vi "XYQuickView.vi"(9 "listOfProfiles":path[](array[path])) -> ()   [LabVIEW 2014]
uses:
  <vilib>/Utility/file.llb/Read From Spreadsheet File (DBL).vi
panel:
  out "XY Graph":cluster{"Y":dbl[], "Y":dbl[]}[](graph)
  in  "fileDelimiter":u16(ring) items=["tab", "space", "comma"]
  in  "open files":bool
  in  "plotType":u16(ring) items=["symbols", "line", "line+symbols"]
  in  "stop":bool
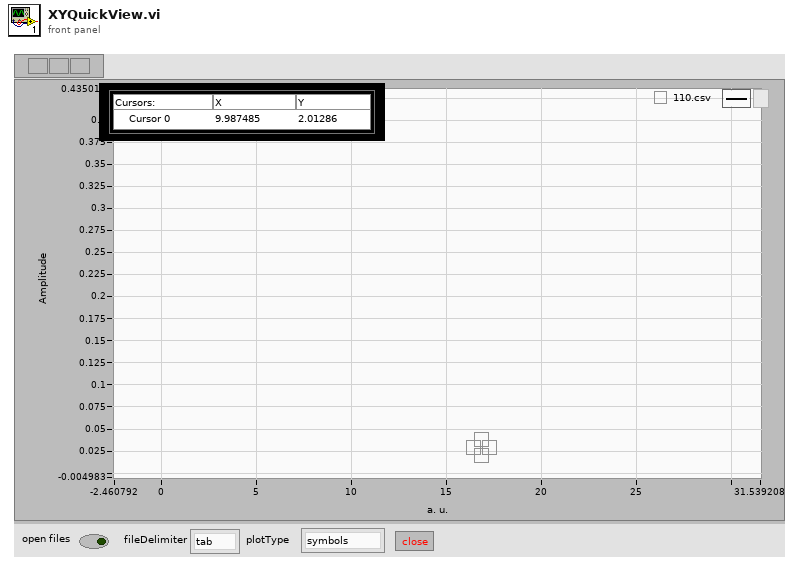
[diagram p1: front panel]
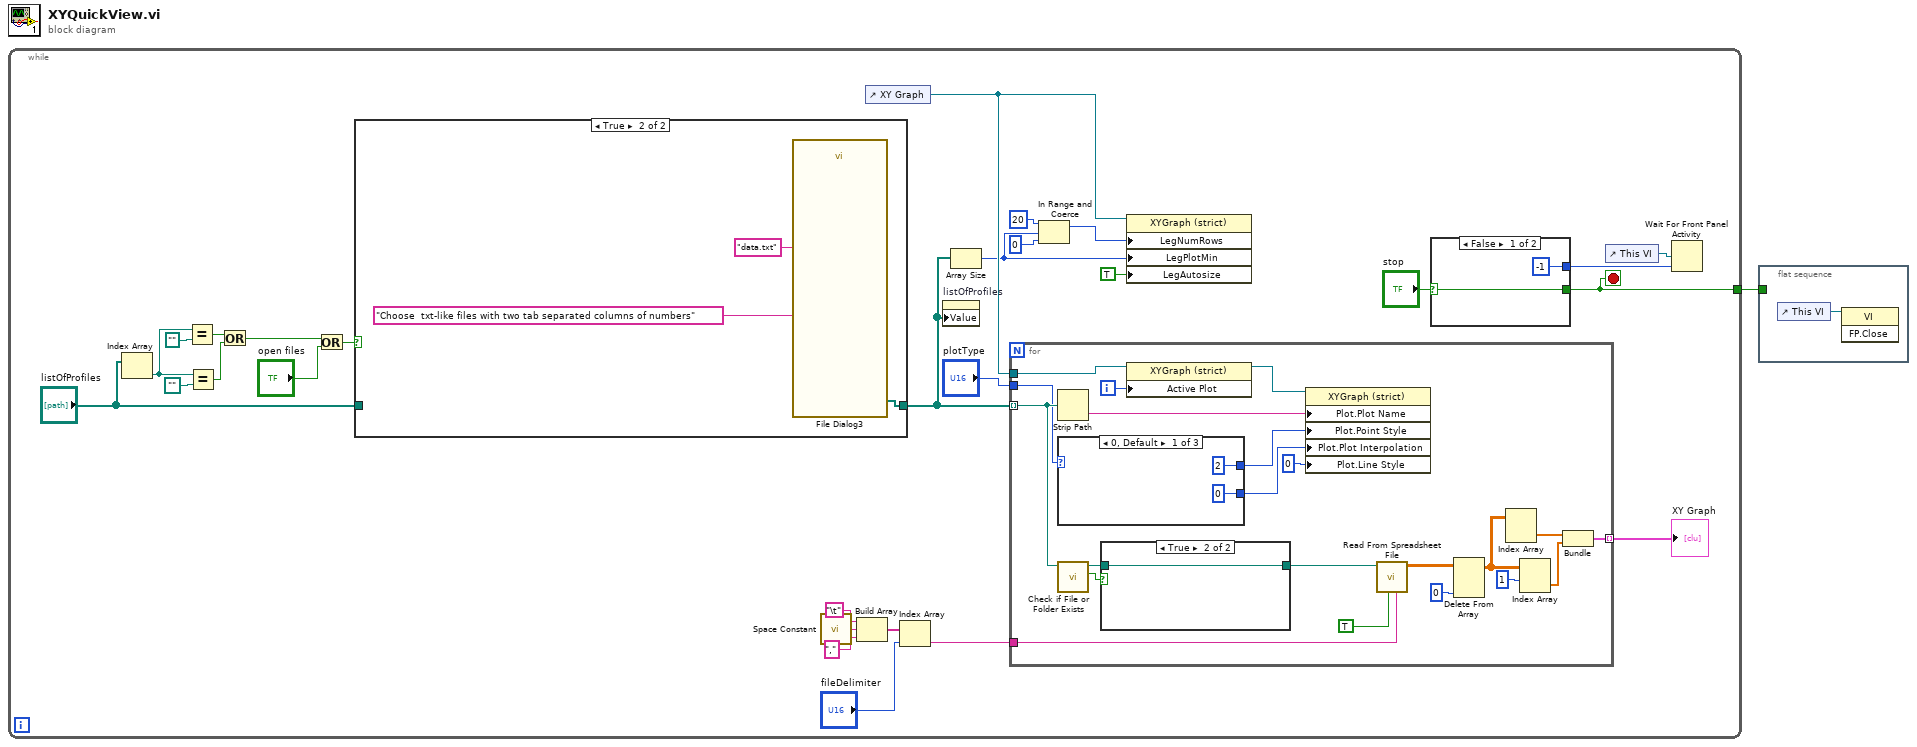
[diagram p0: block diagram]
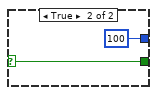
[diagram p3: hidden frame]
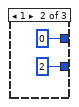
[diagram p4: hidden frame]
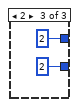
[diagram p5: hidden frame]
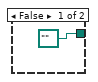
[diagram p6: hidden frame]
diagram:
  n1 = while {
    tunnel: [w17] -> w1
    stop <- w17 stop-if-true
    n2 = Index Array(array="listOfProfiles") -> (element=w20:path)  [unwired: 1 in]
    n3 = Equal?(x=w20, y=path "") -> (x = y?=w22:bool)
    n4 = Equal?(x=w20, y=path "") -> (x = y?=w21:bool)
    n5 = Or(x=w22, y=w21) -> (x .or. y?=w16:bool)
    n6 = Or(x=w16, y="open files") -> (x .or. y?=w14:bool)
    n7 = case shown="True" w14 {
      tunnel: [w30 w31] -> w18
      tunnel: "listOfProfiles" -> [w30 _]
      frame False {
      }
      frame True {
        n8 = call "File Dialog3"("prompt"="Choose  txt-like files with two tab separated columns of numbers" ("Prompt"), "default name"="data.txt") -> ("selected paths"=w31:path[])  [unwired: 10 in, 3 out]
      }
    }
    n9 = call <vilib>:"Space Constant.vi"() -> ("String"=w7:string)
    n10 = Build Array("\t", w7, ",") -> (w11:string[])
    n11 = control-ref of="XY Graph"() -> (w29:refnum<vi>)
    n12 = Index Array(array=w11, index="fileDelimiter") -> (element=w9:string)
    n13 = property on="listOfProfiles" class="Arr (strict)"("Value"=w18) -> ()  [unwired: 2 in, 2 out]
    n14 = Array Size(array=w18) -> (size(s)=w2:i32)
    n15 = for {
      tunnel: w18 -> [w46] mode=indexing
      tunnel: w29 -> [w53]
      tunnel: "plotType" -> [w41]
      tunnel: [w43] -> w12 mode=indexing
      tunnel: w9 -> [w42]
      i -> [w50]
      n16 = Strip Path(path=w46) -> (name=w51:string)  [unwired: 1 out]
      n17 = case shown="0, Default" w41 {
        tunnel: [u8 2 ("Plot.Point Style") 0 2 ("Plot.Point Style")] -> w40
        tunnel: [0 2 2] -> w39
        frame 0, Default {
        }
        frame 1 {
        }
        frame 2 {
        }
      }
      n18 = call <vilib>:"Check if File or Folder Exists.vi"("path"=w46) -> ("file or folder exists?"=w56:bool, "dup path"=w55:path)  [unwired: 8 in, 1 out]
      n19 = case shown="True" w56 {
        tunnel: w55 -> [_ w66]
        tunnel: [path "" ("dup path") w66] -> w54
        frame False {
        }
        frame True {
        }
      }
      n20 = property on="Property Node" class="XYGraph (strict)"(reference=w53, "Active Plot"=w50) -> (reference out=w52:refnum<vi>)  [unwired: 1 in, 1 out]
      n21 = property class="XYGraph (strict)"(reference=w52, "Plot.Plot Name"=w51, "Plot.Point Style"=w40, "Plot.Plot Interpolation"=w39, "Plot.Line Style"=u8 0) -> ()  [unwired: 1 in, 2 out]
      n22 = call-poly <vilib>:"Read From Spreadsheet File.vi"("delimiter (\\t)"=w42, "transpose (no:F)"=TRUE, "file path (dialog if empty)"=w54) -> ("all rows"=w49:dbl[][])  [unwired: 4 in, 4 out]
      n23 = Delete From Array(array=w49, index (col)=0 ("disabled index (col)")) -> (array with subset deleted=w48:dbl[][])  [unwired: 2 in, 1 out]
      n24 = Index Array(array=w48) -> (element=w45:dbl[])  [unwired: 2 in]
      n25 = Index Array(array=w48, index (row)=1) -> (element=w44:dbl[])  [unwired: 1 in]
      n26 = Bundle("all rows"=w45, "all rows"=w44) -> (w43:cluster{"all rows":dbl[], "all rows":dbl[]})  [unwired: 1 in]
    }
    "XY Graph" <- w12
    n27 = In Range and Coerce(upper limit=20, x=w2, lower limit=0) -> (coerced(x)=w3:i32)  [unwired: 1 out]
    n28 = property class="XYGraph (strict)"(reference=w29, "LegNumRows"=w3, "LegPlotMin"=w2, "LegAutosize"=TRUE ("Legend:Autosize")) -> ()  [unwired: 1 in, 2 out]
    n29 = case shown="False" "stop" {
      selector: "stop" -> [w34 w36]
      tunnel: [-1 ("timeout ms (-1 never timeout)") 100 ("timeout ms (-1 never timeout)")] -> w27
      tunnel: [w34 w36] -> w17
      frame False {
      }
      frame True {
      }
    }
    n30 = control-ref of="This VI"() -> (w13:refnum<vi>)
    n31 = Wait For Front Panel Activity(1:w27, 2:w13) -> ()  [unwired: 1 in, 1 out]
  }
  n32 = flat-sequence {
    tunnel: w1 -> [_]
    frame #0 {
      n33 = control-ref of="This VI"() -> (w67:refnum<vi>)
      n34 = invoke class="VI" method="FP.Close"(reference=w67) -> ()  [unwired: 2 in, 3 out]
    }
  }
